vi "kvCanIoCtlSetTxAck.vi"(2 "error in (no error)":errorcluster, 3 "Transmit Ack":enum16{"Off", "On", "Driver Tx Ack Off"}(ring), 4 "Channel Handle (input only)":i32) -> (0 "error out":errorcluster, 1 "Channel Handle (ouput only)":i32)   [LabVIEW 2022 SP3]
doc: "Set Transmit Ack:\n\nTransmit Acknowledges off.\n\nTransmit Acknowledges on.\n\nDriver Transmit Acknowledges Off: Turns off tx ack even for the driver's internal usage. This might enhance performance but will cause some other APIs to stop working (for example, the current size of the transmit queue can not be read when this mode is active.)\n\nThe default value is Transmit Acknowledge off."
uses:
  canlib32.dll
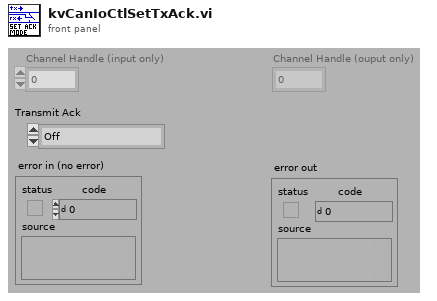
[diagram p1: front panel]
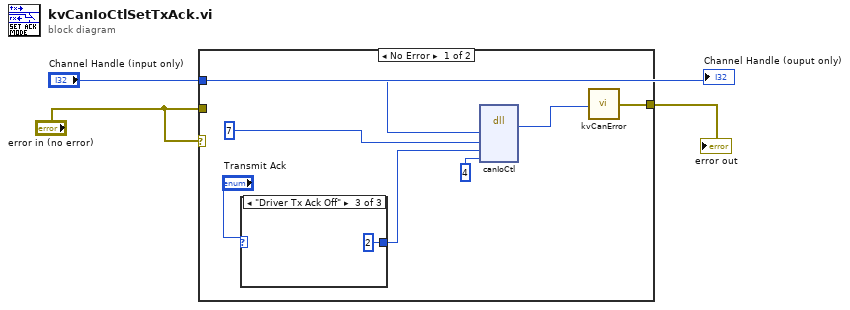
[diagram p0: block diagram]
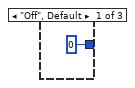
[diagram p2: hidden frame]
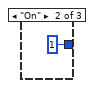
[diagram p3: hidden frame]
diagram:
  n1 = case shown="No Error" "error in (no error)" {
    tunnel: [w10 w14] -> w3
    tunnel: "error in (no error)" -> [_ w14]
    tunnel: "Channel Handle (input only)" -> [w8 _]
    frame No Error {
      n2 = case shown="\"Driver Tx Ack Off\"" "Transmit Ack" {
        tunnel: [0 1 2] -> w4
        frame "Off", Default {
        }
        frame "On" {
        }
        frame "Driver Tx Ack Off" {
        }
      }
      n3 = dll-call lib="canlib32.dll" fn="canIoCtl" label="Call canIoCtl"("handle"=w8, "func"=7, "buf"=w4, "buflen"=4) -> (w9:i32)  [unwired: 7 in, 2 out]
      n4 = call "kvCanError.vi"("error code"=w9) -> ("error out"=w10:errorcluster)
    }
    frame Error {
    }
  }
  "error out" <- w3
  "Channel Handle (ouput only)" <- "Channel Handle (input only)"
